vi "Output Alive.vi"(8 "error in (no error)":errorcluster, 11 "output_request_poller in":refnum<class "output_poller.lvclass">) -> (0 "error out":errorcluster, 2 "alive":bool, 3 "output_request_poller out":refnum<class "output_poller.lvclass">)   [LabVIEW 2015, in "output_poller.lvclass"]
uses:
  output_poller.lvclass
  output_poller.lvclass/output_poller.ctl
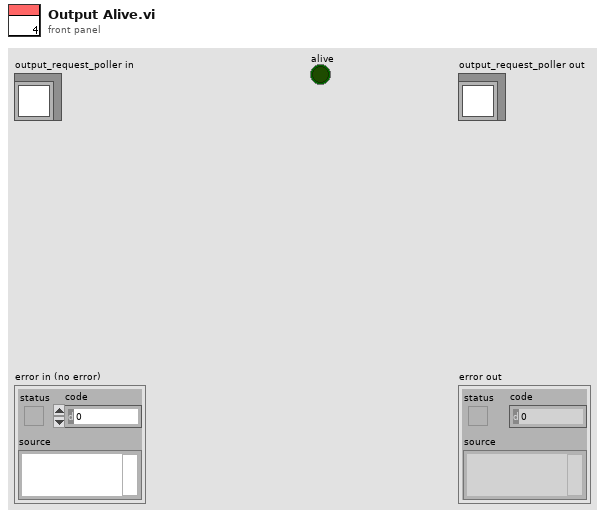
[diagram p1: front panel]
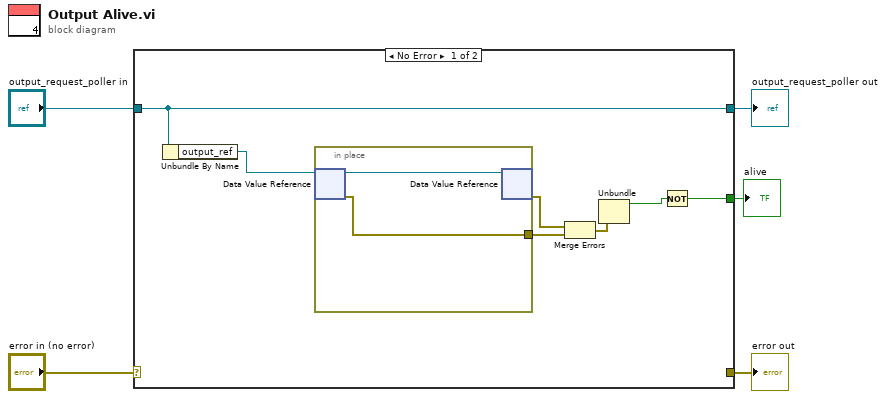
[diagram p0: block diagram]
diagram:
  n1 = case shown="No Error" "error in (no error)" {
    selector: "error in (no error)" -> [_ w16]
    tunnel: [_ w16] -> w4
    tunnel: [w12 w15] -> w2
    tunnel: "output_request_poller in" -> [w12 w15]
    tunnel: [w6 _] -> w1
    frame No Error {
      n2 = Unbundle By Name(w12) -> ("output_ref"=w11:refnum<data-value>)
      n3 = in-place {
        in-place-border: [w13] -> w9
        n4 = in-place-dvr #1(w11) -> (w14:refnum<class "Output.lvclass">, w13:errorcluster)
        n5 = in-place-dvr #1(w14) -> (w10:errorcluster)  [unwired: 1 out]
      }
      n6 = Merge Errors(w10, w9) -> (w8:errorcluster)
      n7 = Unbundle(w8) -> ("status"=w7:bool)  [unwired: 2 out]
      n8 = Not(x=w7) -> (.not. x?=w6:bool)
    }
    frame Error {
    }
  }
  "error out" <- w4
  "output_request_poller out" <- w2
  "alive" <- w1
